vi "sub_SDR_siso_equalizer.vi"(10 "Symbols/Pilot":i32, 11 "In frame":cdb[](array[numeric])) -> (3 "Out Frame":cdb[](array[numeric]))   [LabVIEW 2012]
uses:
  <vilib>/Analysis/2dsp.llb/Decimate (single shot, CDB).vi
  <vilib>/Analysis/NI_AALPro.lvlib
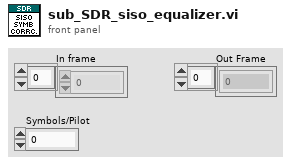
[diagram p1: front panel]
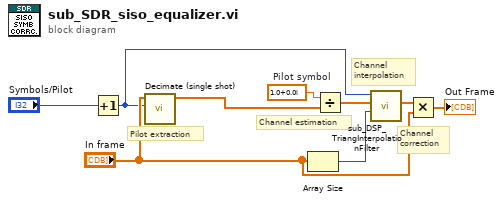
[diagram p0: block diagram]
diagram:
  w2 = cdb 1.0+0.0i  # Pilot symbol
  # "Channel\ncorrection"
  # "Channel\ninterpolation"
  # "Channel estimation"
  # "Pilot extraction"
  n1 = Increment(x="Symbols/Pilot") -> (x+1=w4:i32)
  n2 = call-poly <vilib>:"Decimate (single shot).vi"("decimating factor"=w4, "X"="In frame") -> ("Decimated Array"=w1:cdb[])  [unwired: 8 in, 1 out]
  n3 = Array Size(array="In frame") -> (size(s)=w5:i32)
  n4 = Divide(x=w2, y=w1) -> (x/y=w3:cdb[])
  n5 = call "sub_DSP_TriangInterpolationFilter.vi"("Desired Len"=w5, "X"=w3, "Interpolation factor"=w4) -> ("Interpolated X"=w7:cdb[])  [unwired: 8 in]
  n6 = Multiply(x=w7, y="In frame") -> (x*y=→"Out Frame":cdb[])
